vi "Read Attributes.vi"(11 "Abstract Message Template in":refnum<class "String Data Msg.lvclass">) -> (2 "Payload":cluster{"String":string}, 3 "Abstract Message Template out":refnum<class "String Data Msg.lvclass">)   [LabVIEW 2020, in "String Data Msg.lvclass"]
uses:
  String Data Msg.lvclass
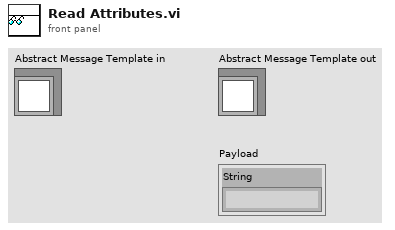
[diagram p1: front panel]
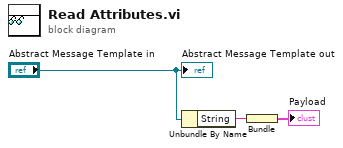
[diagram p0: block diagram]
diagram:
  n1 = Unbundle By Name("Abstract Message Template in") -> ("String"=w1:string)
  n2 = Bundle("String"=w1) -> (→"Payload":cluster{"String":string})  [unwired: 1 in]
  "Abstract Message Template out" <- "Abstract Message Template in"
